vi "rosbridge.vi"() -> ()   [LabVIEW 2015, in "Biblioteka moduł map v3.lvlib" / "ROS.lvlib"]
uses:
  ROS.lvlib
  Zmienne/szablon odometry_filtered_local.ctl
  Gobal for ROS.vi
  Zmienne/Lokalizacja GPS/longitude.vi
  Zmienne/Lokalizacja GPS/latitude.vi
  Zmienne/szablon odometry_filtered_local.vi
  <vilib>/Intelligent Energy/WebSockets API/WebSockets/WebSockets.lvlib
  Zmienne/Zmienne.lvlib
  Zmienne/Lokalizacja GPS/Lokalizacja GPS.lvlib
panel:
  out "value":T1
  out "ROS data IMU 2":T2={"topic"="", "msg"={"header"={"seq"=63049, "stamp"={"secs"=0, "nsecs"=0}, "frame_id"="imu_link"}, "orientation"={"x"=0.0, "y"=0.0, "z"=0.0, "w"=0.0}, "orientation_covariance"=[], "angular_velocity"={"x"=0.0, "y"=0.0, "z"=0.0}, "angular_velocity_covariance"=[], "linear_acceleration"={"x"=0.0, "y"=0.0, "z"=0.0}, "linear_acceleration_covariance"=[]}, "op"=""}
  in  "Tab Control":enum32{"GPS Łazik", "Odometria Łazik", "ERL "}(tab)
  out "ROS data read 4":T3
  in  "ROSB READ":bool
  in  "Topic string":string="{ \"op\": \"subscribe\", \"topic\" : \"/fix\" }"
  in  "STOP ROS READ":bool
  out "raw frame":string
  in  "ROS data read 3":T3
  out "error out 2":errorcluster
  in  "ROSB READ 2":bool
  in  "Topic string 2":string="{ \"op\": \"subscribe\", \"topic\" : \"/odometry/filtered/local\" }"
  out "error out 3":errorcluster
  out "raw frame 2":string
  in  "STOP ROS READ 2":bool
  in  "szablon odometry/filtered/local":T4
  out "szablon odometry/filtered/local 2":T4
  in  "Cluster":T1
  in  "ROSB READ 3":bool
  in  "Topic string 3":string="{ \"op\": \"subscribe\", \"topic\" : \"/fix\" }"
  out "error out 4":errorcluster
  in  "STOP ROS READ 3":bool
  out "raw frame 3":string
  out "x-y":u32
  in  "ROS data IMU":T2={"topic"="", "msg"={"header"={"seq"=63049, "stamp"={"secs"=0, "nsecs"=0}, "frame_id"="imu_link"}, "orientation"={"x"=0.0, "y"=0.0, "z"=0.0, "w"=0.0}, "orientation_covariance"=[], "angular_velocity"={"x"=0.0, "y"=0.0, "z"=0.0}, "angular_velocity_covariance"=[], "linear_acceleration"={"x"=0.0, "y"=0.0, "z"=0.0}, "linear_acceleration_covariance"=[]}, "op"=""}
  # "Topic /fix na gpsa \ntopic rio/odom na prędkości\nIMU /data"
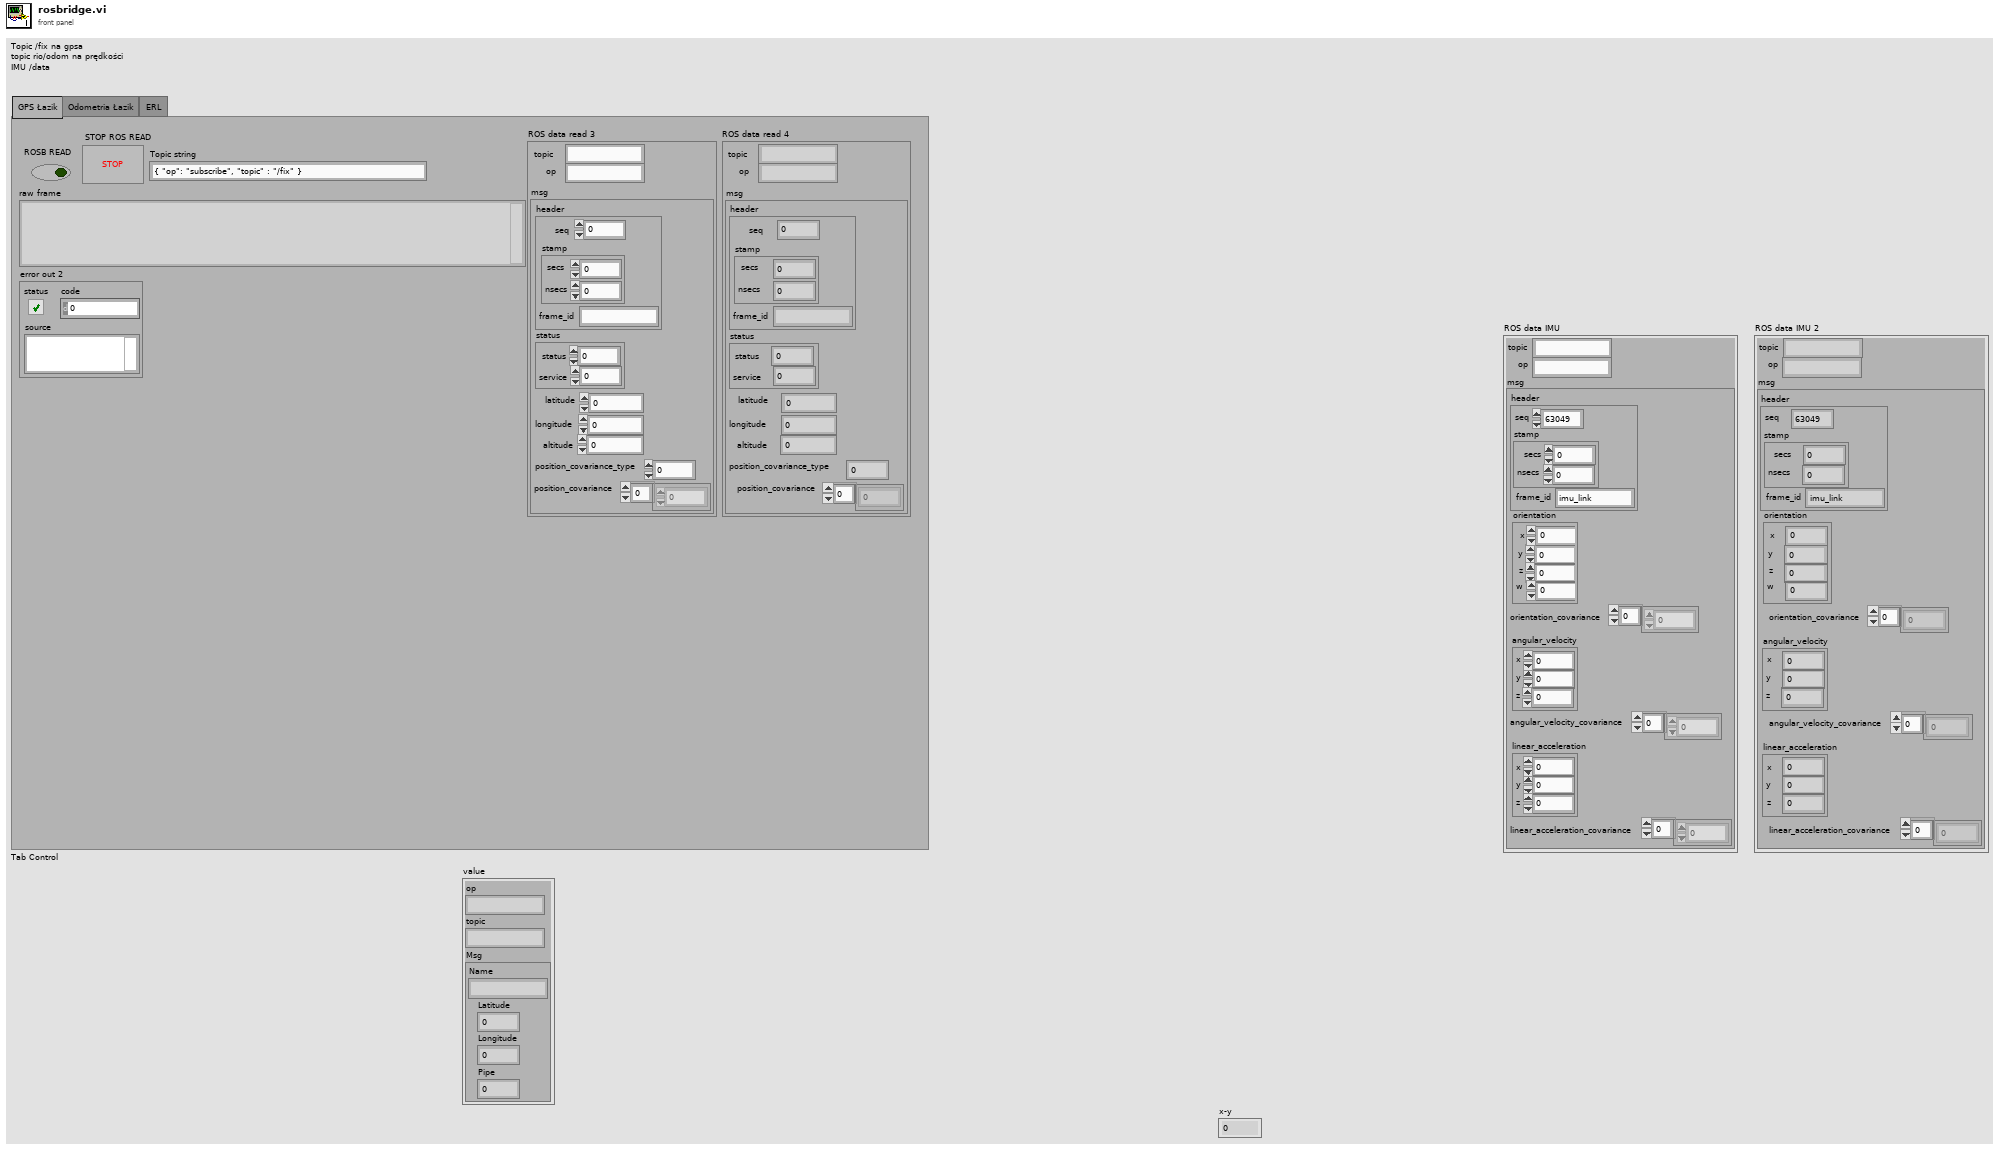
[diagram p1: front panel]
types:
  T1 = cluster{"op":string, "topic":string, "Msg":cluster{"Name":string, "Latitude":dbl, "Longitude":dbl, "Pipe":dbl}}
  T2 = cluster{"topic":string, "msg":cluster{"header":cluster{"seq":u32, "stamp":cluster{"secs":u32, "nsecs":i32}, "frame_id":string}, "orientation":cluster{"x":dbl, "y":dbl, "z":dbl, "w":dbl}, "orientation_covariance":dbl[], "angular_velocity":cluster{"x":dbl, "y":dbl, "z":dbl}, "angular_velocity_covariance":dbl[], "linear_acceleration":cluster{"x":dbl, "y":dbl, "z":dbl}, "linear_acceleration_covariance":dbl[]}, "op":string}
  T3 = cluster{"topic":string, "msg":cluster{"header":cluster{"seq":u32, "stamp":cluster{"secs":u32, "nsecs":i32}, "frame_id":string}, "status":cluster{"status":u32, "service":i32}, "position_covariance":dbl[], "latitude":dbl, "longitude":dbl, "altitude":i32, "position_covariance_type":dbl}, "op":string}
  T4 = typedef "Biblioteka moduł map v3.lvlib/Zmienne.lvlib/szablon odometry_filtered_local.ctl" = cluster{"topic":string, "msg":cluster{"header":cluster{"seq":u32, "stamp":cluster{"secs":u32, "nsecs":i32}, "frame_id":string}, "child_frame_id":string, "pose":cluster{"pose":cluster{"position":cluster{"y":dbl, "z":dbl, "x":dbl}, "orientation":cluster{"y":dbl, "z":dbl, "x":dbl, "w":dbl}}, "covariance":dbl[]}, "twist":cluster{"twist":cluster{"linear":cluster{"y":dbl, "z":dbl, "x":dbl}, "angular":cluster{"y":dbl, "z":dbl, "x":dbl}}, "covariance":dbl[]}}, "op":string}
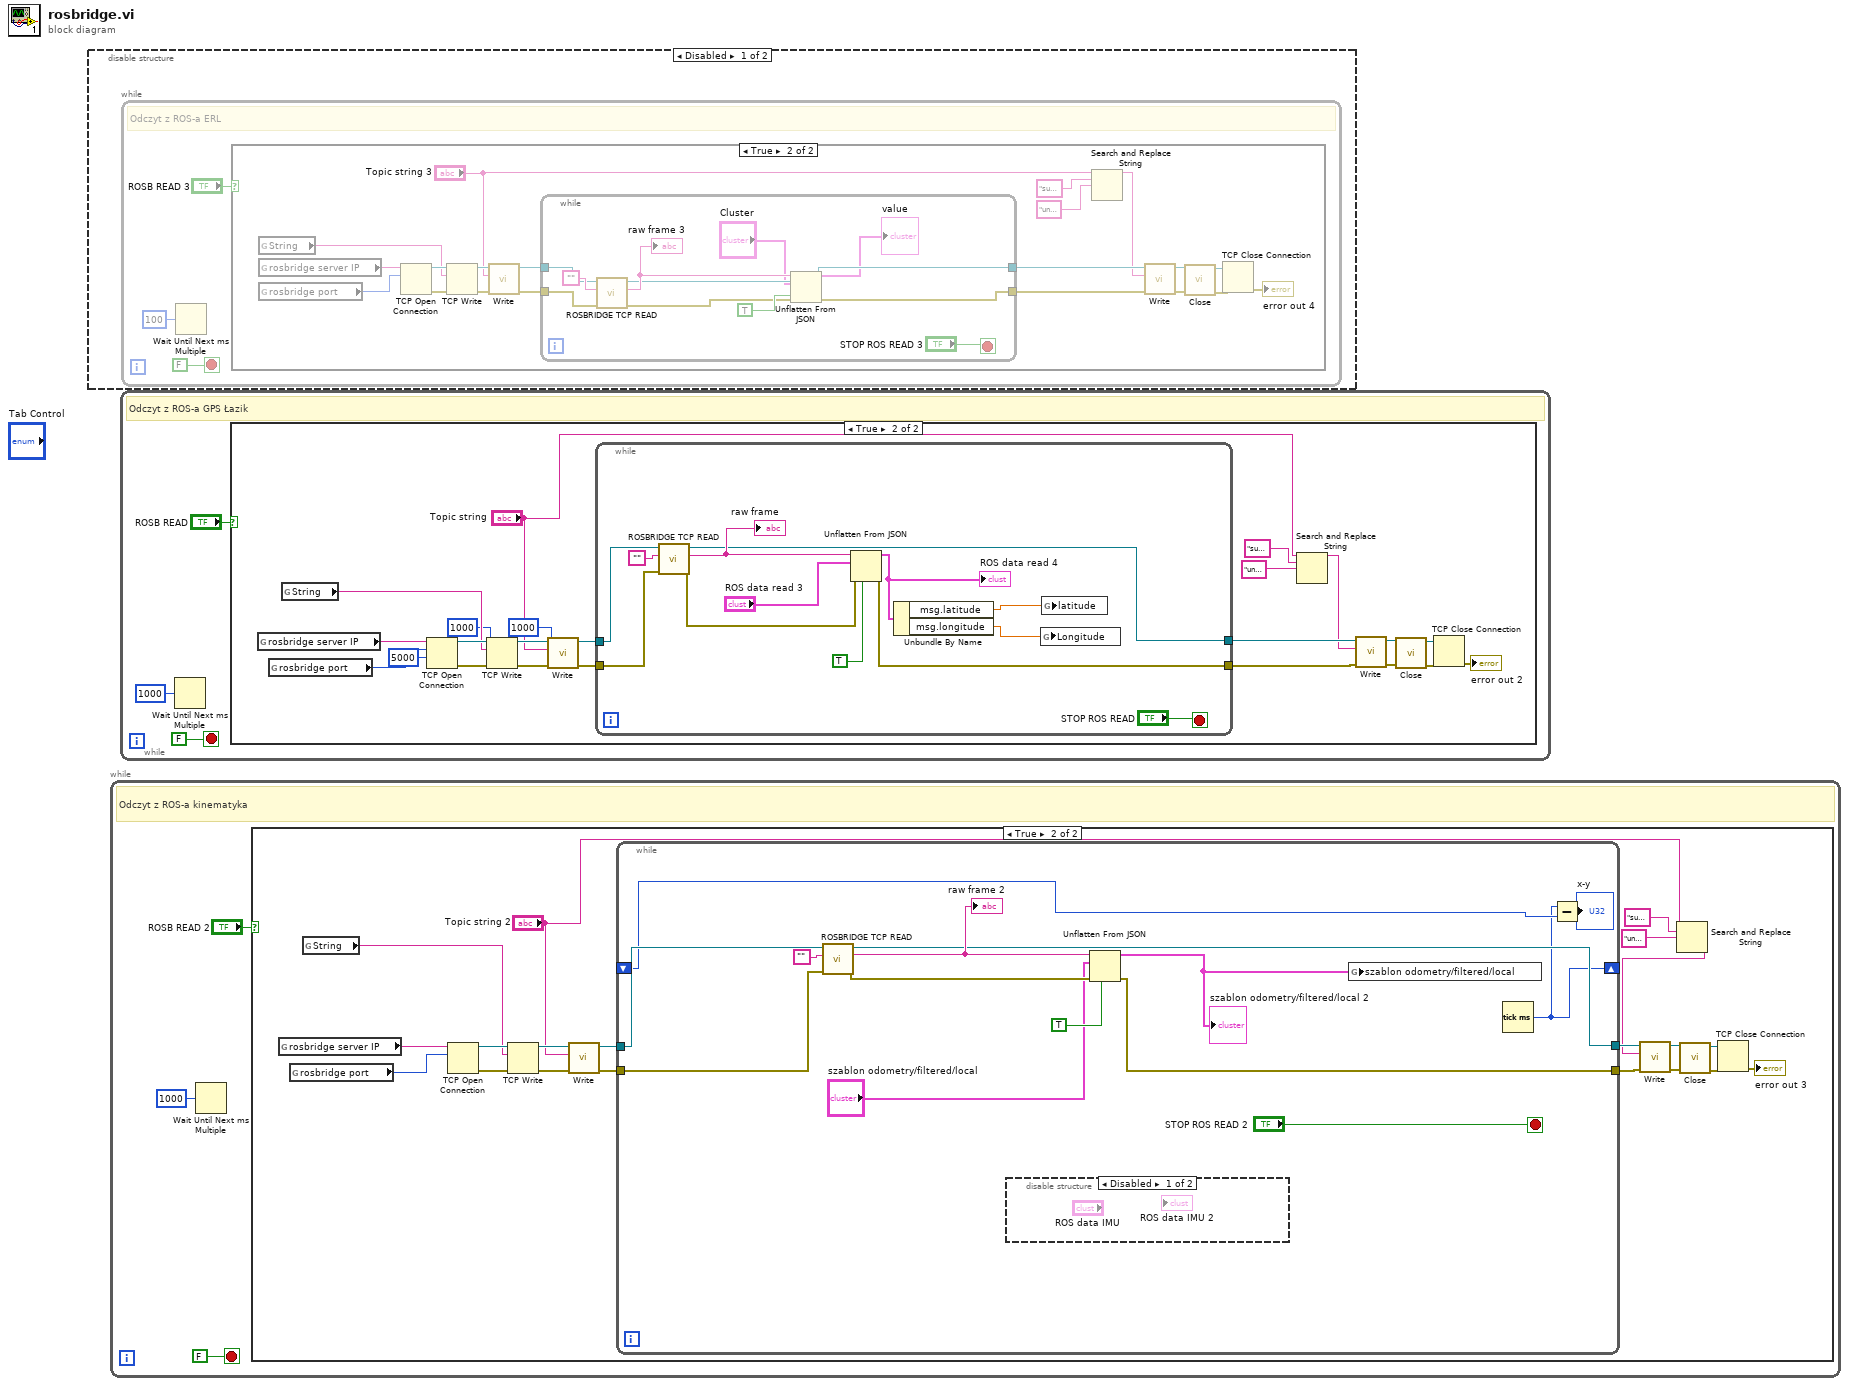
[diagram p0: block diagram]
diagram:
  n1 = disable-structure shown="Disabled" {
    frame Disabled {
      n2 = while {
        stop <- FALSE stop-if-true
        # "Odczyt z ROS-a ERL"
        n3 = Wait Until Next ms Multiple(millisecond multiple=u32 100 ("milliseconds to wait")) -> ()  [unwired: 1 out]
        n4 = case shown="True" "ROSB READ 3" {
          frame False {
          }
          frame True {
            n5 = global read "Gobal for ROS.vi" "String"() -> (w14:string)
            n6 = global read "Gobal for ROS.vi" "rosbridge server IP"() -> (w13:string)
            n7 = global read "Gobal for ROS.vi" "rosbridge port"() -> (w12:u16)
            n8 = TCP Open Connection(address=w13, remote port or service name=w12) -> (connection ID=w23:refnum<k5>, error out=w22:errorcluster)  [unwired: 3 in]
            n9 = TCP Write(connection ID=w23, data in=w14, error in (no error)=w22) -> (connection ID out=w19:refnum<k5>, error out=w18:errorcluster)  [unwired: 1 in, 1 out]
            n10 = call <vilib>:"Write.vi"("error in (no error)"=w18, "Data"="Topic string 3", "WebSocket Connection in"=w19) -> ("error out"=w16:errorcluster, "WebSocket Connection out"=w17:refnum<k5>)  [unwired: 7 in]
            n11 = while {
              tunnel: [w27] -> w9
              tunnel: [w34] -> w8
              tunnel: w17 -> [w29]
              tunnel: w16 -> [w28]
              stop <- "STOP ROS READ 3" stop-if-true
              n12 = call "ROSBRIDGE TCP READ.vi"("error in (no error)"=w28, "String in"="", "TCP Network Connection in"=w29) -> ("error out"=w26:errorcluster, "String out"=w30:string, "TCP Network Connection out"=w27:refnum<k5>)  [unwired: 6 in]
              "raw frame 3" <- w30
              n13 = Unflatten From JSON(JSON string=w30, type and defaults="Cluster", default null elements? (F)=TRUE, error in (no error)=w26) -> (value=→"value":T1, error out=w34:errorcluster)  [unwired: 3 in]
            }
            n14 = Search and Replace String(input string="Topic string 3", search string="subscribe", replace string="unsubscribe" ("search string")) -> (result string=w7:string)  [unwired: 5 in, 3 out]
            n15 = call <vilib>:"Write.vi"("error in (no error)"=w8, "Data"=w7, "WebSocket Connection in"=w9) -> ("error out"=w10:errorcluster, "WebSocket Connection out"=w11:refnum<k5>)  [unwired: 7 in]
            n16 = call <vilib>:"Close.vi"("error in (no error)"=w10, "WebSocket Connection in"=w11) -> ("error out"=w20:errorcluster, "WebSocket Connection in"=w21:refnum<k5>)  [unwired: 8 in]
            n17 = TCP Close Connection(connection ID=w21, error in (no error)=w20) -> (error out=→"error out 4":errorcluster)  [unwired: 1 in, 1 out]
          }
        }
      }
    }
    frame Enabled {
    }
  }
  n18 = while {
    stop <- FALSE stop-if-true
    # "Odczyt z ROS-a kinematyka"
    n19 = Wait Until Next ms Multiple(millisecond multiple=u32 1000 ("milliseconds to wait")) -> ()  [unwired: 1 out]
    n20 = case shown="True" "ROSB READ 2" {
      frame False {
      }
      frame True {
        n21 = global read "Gobal for ROS.vi" "rosbridge server IP"() -> (w47:string)
        n22 = global read "Gobal for ROS.vi" "rosbridge port"() -> (w46:u16)
        n23 = global read "Gobal for ROS.vi" "String"() -> (w48:string)
        n24 = TCP Open Connection(address=w47, remote port or service name=w46) -> (connection ID=w57:refnum<k5>, error out=w56:errorcluster)  [unwired: 3 in]
        n25 = TCP Write(connection ID=w57, data in=w48, error in (no error)=w56) -> (connection ID out=w53:refnum<k5>, error out=w52:errorcluster)  [unwired: 1 in, 1 out]
        n26 = call <vilib>:"Write.vi"("error in (no error)"=w52, "Data"="Topic string 2", "WebSocket Connection in"=w53) -> ("error out"=w50:errorcluster, "WebSocket Connection out"=w51:refnum<k5>)  [unwired: 7 in]
        n27 = while {
          tunnel: [w64] -> w43
          tunnel: [w71] -> w42
          tunnel: w51 -> [w66]
          tunnel: w50 -> [w65]
          shift-right: [w59] -> _
          shift-left: _ -> [w60]
          stop <- "STOP ROS READ 2" stop-if-true
          n28 = call "ROSBRIDGE TCP READ.vi"("error in (no error)"=w65, "String in"="", "TCP Network Connection in"=w66) -> ("error out"=w63:errorcluster, "String out"=w67:string, "TCP Network Connection out"=w64:refnum<k5>)  [unwired: 6 in]
          "raw frame 2" <- w67
          n29 = disable-structure shown="Disabled" {
            frame Disabled {
            }
            frame Enabled {
            }
          }
          n30 = Unflatten From JSON(JSON string=w67, type and defaults="szablon odometry/filtered/local", default null elements? (F)=TRUE, error in (no error)=w63) -> (value=w58:T4, error out=w71:errorcluster)  [unwired: 3 in]
          "szablon odometry/filtered/local 2" <- w58
          n31 = global write "szablon odometry_filtered_local.vi" "szablon odometry/filtered/local"(w58) -> ()
          n32 = Tick Count (ms)() -> (millisecond timer value=w59:u32)
          n33 = Subtract(x=w59, y=w60) -> (x-y=→"x-y":u32)
        }
        n34 = Search and Replace String(input string="Topic string 2", search string="subscribe", replace string="unsubscribe" ("search string")) -> (result string=w41:string)  [unwired: 5 in, 3 out]
        n35 = call <vilib>:"Write.vi"("error in (no error)"=w42, "Data"=w41, "WebSocket Connection in"=w43) -> ("error out"=w44:errorcluster, "WebSocket Connection out"=w45:refnum<k5>)  [unwired: 7 in]
        n36 = call <vilib>:"Close.vi"("error in (no error)"=w44, "WebSocket Connection in"=w45) -> ("error out"=w54:errorcluster, "WebSocket Connection in"=w55:refnum<k5>)  [unwired: 8 in]
        n37 = TCP Close Connection(connection ID=w55, error in (no error)=w54) -> (error out=→"error out 3":errorcluster)  [unwired: 1 in, 1 out]
      }
    }
  }
  n38 = while {
    stop <- FALSE stop-if-true
    # "Odczyt z ROS-a GPS Łazik"
    n39 = Wait Until Next ms Multiple(millisecond multiple=u32 1000 ("milliseconds to wait")) -> ()  [unwired: 1 out]
    n40 = case shown="True" "ROSB READ" {
      frame False {
      }
      frame True {
        n41 = global read "Gobal for ROS.vi" "rosbridge server IP"() -> (w87:string)
        n42 = global read "Gobal for ROS.vi" "rosbridge port"() -> (w86:u16)
        n43 = global read "Gobal for ROS.vi" "String"() -> (w88:string)
        n44 = TCP Open Connection(address=w87, remote port or service name=w86, timeout ms (60000)=5000) -> (connection ID=w97:refnum<k5>, error out=w96:errorcluster)  [unwired: 2 in]
        n45 = TCP Write(connection ID=w97, data in=w88, error in (no error)=w96, 9:1000 ("timeout ms (25000)")) -> (connection ID out=w93:refnum<k5>, error out=w92:errorcluster)  [unwired: 1 out]
        n46 = call <vilib>:"Write.vi"("error in (no error)"=w92, "timeout ms (5000)"=1000, "Data"="Topic string", "WebSocket Connection in"=w93) -> ("error out"=w90:errorcluster, "WebSocket Connection out"=w91:refnum<k5>)  [unwired: 6 in]
        n47 = while {
          tunnel: [w103] -> w83
          tunnel: [w110] -> w82
          tunnel: w91 -> [w105]
          tunnel: w90 -> [w104]
          stop <- "STOP ROS READ" stop-if-true
          n48 = call "ROSBRIDGE TCP READ.vi"("error in (no error)"=w104, "String in"="", "TCP Network Connection in"=w105) -> ("error out"=w102:errorcluster, "String out"=w106:string, "TCP Network Connection out"=w103:refnum<k5>)  [unwired: 6 in]
          "raw frame" <- w106
          n49 = Unflatten From JSON(JSON string=w106, type and defaults="ROS data read 3", default null elements? (F)=TRUE, error in (no error)=w102) -> (value=w98:T3, error out=w110:errorcluster)  [unwired: 3 in]
          "ROS data read 4" <- w98
          n50 = Unbundle By Name(w98) -> ("msg.latitude"=w100:dbl, "msg.longitude"=w99:dbl)
          n51 = global write "longitude.vi" "Longitude"(w99) -> ()
          n52 = global write "latitude.vi" "latitude"(w100) -> ()
        }
        n53 = Search and Replace String(input string="Topic string", search string="subscribe", replace string="unsubscribe" ("search string")) -> (result string=w81:string)  [unwired: 5 in, 3 out]
        n54 = call <vilib>:"Write.vi"("error in (no error)"=w82, "Data"=w81, "WebSocket Connection in"=w83) -> ("error out"=w84:errorcluster, "WebSocket Connection out"=w85:refnum<k5>)  [unwired: 7 in]
        n55 = call <vilib>:"Close.vi"("error in (no error)"=w84, "WebSocket Connection in"=w85) -> ("error out"=w94:errorcluster, "WebSocket Connection in"=w95:refnum<k5>)  [unwired: 8 in]
        n56 = TCP Close Connection(connection ID=w95, error in (no error)=w94) -> (error out=→"error out 2":errorcluster)  [unwired: 1 in, 1 out]
      }
    }
  }
